vi "Clear Hardware.vi"(2 "error in (no error)":errorcluster, 3 "TestMenu in":refnum<class "TestMenu.lvclass">) -> (0 "error out":errorcluster, 1 "TestMenu out":refnum<class "TestMenu.lvclass">)   [LabVIEW 2013, in "TestMenu.lvclass"]
doc: "This VI resets any necessary hardware so that the device will be ready for the next run."
uses:
  TestMenu.lvclass
  Device/Device.lvclass
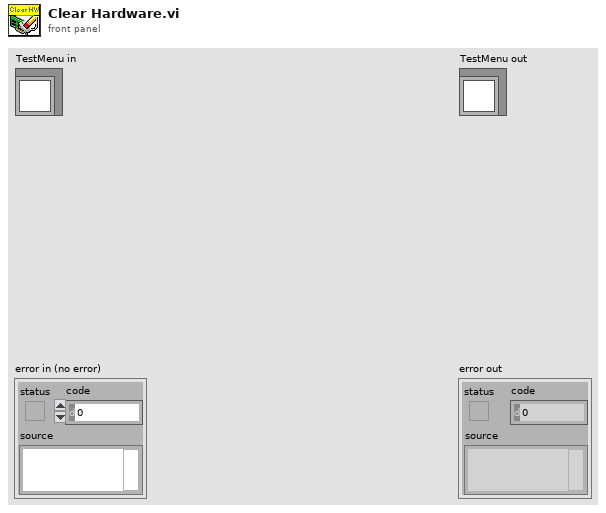
[diagram p1: front panel]
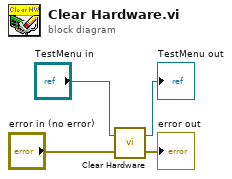
[diagram p0: block diagram]
diagram:
  n1 = call-parent "Clear Hardware.vi"("error in (no error)"="error in (no error)", "Device in"="TestMenu in") -> ("error out"=→"error out":errorcluster, "Device out"=→"TestMenu out":refnum<class "TestMenu.lvclass">)
